vi "RWNoise-Init Stimulus.vi"(0 "RW Noise Params":T29, 7 "Expt State":T27, 11 "error in (no error)":errorcluster, 12 "RWN Stim":T28) -> (4 "Runtime":T1={"Stimulus"={"Waveform"={"Type"=enum."Tone", "Tone"={"Frequency (kHz)"=0.0, "Last Freq"=0.0, "Last Phase"=0.0}, "Pulse Train"={"Pulse width (us)"=0.0, "Pulse rate (Hz)"=0.0, "Gap (ms)"=0.0, "Polarity"=enum."POS", "PT State"={"Template"=[], "Nperiod"=0, "Index"=0, "Pulse Rate (Hz)"=0.0, "Phase (cycles)"=0.0, "Noff"=0}, "Asynch"=FALSE}, "Noise"={"InvFilt"=FALSE, "Noise"=[], "CurPt"=0, "Aweight"=FALSE, "Seed"=0, "afile"=path ""}, "File"={"Filename"=path "", "Signal"=[], "Channel"=0, "stream"=FALSE, "offset"=0, "nreps"=0, "loops"=0, "Randomize"=FALSE, "order"=[], "Seed"=0, "Tokens"=0}, "FMSweep"={"Rate (oct/s)"=0.0, "Fmin (Hz)"=0.0, "Fmax (Hz)"=0.0, "Ramp (ms)"=0.0, "Linear"=FALSE}, "Chirp Train"={"Params"={"Fmin (kHz)"=4.0, "Fmax (kHz)"=64.0, "Compensate"=FALSE, "Duration (ms)"=2.0}, "Data"={"WF"=[]}}, "Complex Tone"={"Params"={"F0 (Hz)"=0.0, "Band"={"Flow (Hz)"=0.0, "Fhigh (Hz)"=0.0}, "Phase"=enum."Cosine", "Min F0 (Hz)"=0.0, "Max F0 (Hz)"=0.0, "ContinRandPhase"=FALSE, "Max peak factor"=inf, "Max mod depth"=2.0, "MinHarmNum"=0, "MaxHarmNum"=0, "Level Mode"=enum."per component", "% jitter"=0.0}, "Data"={"Ncomp"=0, "MinHarm"=0, "Phase"=[], "Amplitude"=[], "Npts/frame"=0, "Last F0"=0.0, "Fmin"=0.0, "Fmax"=0.0, "Lslope"=0.0, "randphase"=FALSE, "overall rms"=FALSE, "fmult"=[], "jittered"=FALSE}}, "Moving Ripple"={"Params"={"Fmin"=0.0, "Fmax"=0.0, "Density"=0.0, "Velocity"=0.0, "Depth"=0.0, "Phase"=0.0, "Comp/oct"=0}, "Data"={"Freq"=[], "A"=[], "phase"=[], "Phase"=0.0}}}, "Filter"={"Type"=enum."Lowpass", "CF (kHz)"=0.0, "BW (kHz)"=0.0, "Cascade"=FALSE, "Quadrature"=FALSE, "Scale Factor"=0.0, "Stages"=[], "Class"=enum."Elliptic", "Order"=0, "BWUnits"=enum."Linear"}, "Burst"={"Active"=FALSE, "Delay (ms)"=0.0, "Duration (ms)"=0.0, "Ramp (ms)"=0.0, "Rate (Hz)"=0.0, "Trepeat (ms)"=0.0, "Repeat"=FALSE}, "Level"={"Level"=0.0, "Units"=enum."dB atten", "Max"=0.0, "Multiplier"=0.0, "Cal File"=path "", "Cal"={"Freq (Hz)"=[], "Mag (dB SPL)"=[], "Phase (deg)"=[]}}, "Name"="", "Advanced"={"Rep Mask"="", "AltPol"=FALSE, "Var"="", "Expr"="", "Persist"=FALSE}, "SAM"={"Active"=FALSE, "Frequency (Hz)"=0.0, "Depth"=0.0, "Init Phase (cycles)"=0.0, "phase (degrees)"=0.0, "Asynch"=FALSE}}, "Fs (Hz)"=0.0, "AO Npts"=0, "AO Channels"=[], "Active"=FALSE, "AINpts"=0, "WinPts"=0, "NUpdate"=0} {"Stimulus"."Filter"."Stages"."IIR Filter"."Forward Coefficients" format="%.4f"; "Stimulus"."Filter"."Stages"."IIR Filter"."Reverse Coefficients" format="%.4f"}, 8 "Coerced Freq (kHz)":dbl, 10 "Coerced pulse rate (Hz)":dbl, 15 "error out":errorcluster)   [LabVIEW 2020]
uses:
  RWNoise Params.ctl
  epl-vi-lib/Utility VIs/Type Defs/Left-Right ring.ctl
  RWNoise-Stim Params.ctl
  CFTS Main Panel SubVIs/CFTS-Experiment State.ctl
  epl-vi-lib/Signal Synthesis VIs/Controls/Stimulus Channel (Full)/Full Stimulus Channel Data.ctl
  epl-vi-lib/Signal Synthesis VIs/Controls/Waveform XCtl/Waveform Data.ctl
  epl-vi-lib/Signal Synthesis VIs/Controls/Waveform XCtl/Waveform Enum.ctl
  epl-vi-lib/Signal Synthesis VIs/Waveform VIs/Tone VIs/Tone Params.ctl
  epl-vi-lib/Signal Synthesis VIs/Waveform VIs/Pulse Train VIs/Pulse Train Params.ctl
  epl-vi-lib/Signal Synthesis VIs/Waveform VIs/Pulse Train VIs/Pulse Polarity.ctl
  epl-vi-lib/Signal Synthesis VIs/Waveform VIs/Pulse Train VIs/PT-Continuous State.ctl
  epl-vi-lib/Signal Synthesis VIs/Waveform VIs/Noise VIs/Noise Params.ctl
  epl-vi-lib/Signal Synthesis VIs/Waveform VIs/File VIs/StimFile-Params.ctl
  epl-vi-lib/Signal Synthesis VIs/Waveform VIs/FM Sweep VIs/FM Sweep Params.ctl
  epl-vi-lib/Signal Synthesis VIs/Waveform VIs/Chirp Train VIs/Chirp Train.ctl
  epl-vi-lib/Signal Synthesis VIs/Waveform VIs/Chirp Train VIs/Chirp Train Params.ctl
  epl-vi-lib/Signal Synthesis VIs/Waveform VIs/Complex Tone VIs/CT-Params.ctl
  epl-vi-lib/Signal Synthesis VIs/Waveform VIs/Complex Tone VIs/CT-Phase Enum.ctl
  epl-vi-lib/Signal Synthesis VIs/Waveform VIs/Complex Tone VIs/CT-Runtime Data.ctl
  epl-vi-lib/Signal Synthesis VIs/Waveform VIs/Moving Ripple VIs/Moving Ripple.ctl
  epl-vi-lib/Signal Synthesis VIs/Waveform VIs/Moving Ripple VIs/Moving Ripple.Params.ctl
  epl-vi-lib/Signal Synthesis VIs/Waveform VIs/Moving Ripple VIs/Moving Ripple.Data.ctl
  epl-vi-lib/Signal Synthesis VIs/Controls/Advanced Filter XCtl/Filter Data.ctl
  epl-vi-lib/Signal Synthesis VIs/Filter VIs/Filter-Bandwidth Units.ctl
  epl-vi-lib/Signal Synthesis VIs/Controls/Burst XCtl/Burst Data.ctl
  epl-vi-lib/Signal Synthesis VIs/Controls/Level XCtl/Level Data.ctl
  epl-vi-lib/Signal Synthesis VIs/Controls/Level XCtl/Level Units.ctl
  epl-vi-lib/Signal Synthesis VIs/Controls/Advanced Options XCtl/Advanced Stimulus Options.ctl
  epl-vi-lib/Signal Synthesis VIs/Modulation VIs/SAM VIs/SAM Params.ctl
  RWNoise-Runtime Data.ctl
  epl-vi-lib/Connection VIs/Type Defs/Output sources.ctl
  epl-vi-lib/Utility VIs/Type Defs/Speaker ring.ctl
  epl-vi-lib/Signal Synthesis VIs/Top Level VIs/Stimulus-Initialize (full).vi
  epl-vi-lib/Signal Synthesis VIs/Controls/Advanced Filter XCtl/Advanced Filter XCtl.xctl
  epl-vi-lib/Signal Synthesis VIs/Controls/Level XCtl/Level XCtl.xctl
  epl-vi-lib/Signal Synthesis VIs/Controls/Burst XCtl/Burst Control.xctl
  epl-vi-lib/Signal Synthesis VIs/Controls/Waveform XCtl/Waveform XCtl.xctl
  epl-vi-lib/Signal Synthesis VIs/Controls/Advanced Options XCtl/Advanced Stimulus Options.xctl
  epl-vi-lib/Signal Synthesis VIs/Controls/Stimulus Channel (Full)/Stimulus Channel (Full).xctl
panel:
  in  "Stimulus":T2={"Waveform"={"Type"=enum."Tone", "Tone"={"Frequency (kHz)"=0.0, "Last Freq"=0.0, "Last Phase"=0.0}, "Pulse Train"={"Pulse width (us)"=0.0, "Pulse rate (Hz)"=0.0, "Gap (ms)"=0.0, "Polarity"=enum."POS", "PT State"={"Template"=[], "Nperiod"=0, "Index"=0, "Pulse Rate (Hz)"=0.0, "Phase (cycles)"=0.0, "Noff"=0}, "Asynch"=FALSE}, "Noise"={"InvFilt"=FALSE, "Noise"=[], "CurPt"=0, "Aweight"=FALSE, "Seed"=0, "afile"=path ""}, "File"={"Filename"=path "", "Signal"=[], "Channel"=0, "stream"=FALSE, "offset"=0, "nreps"=0, "loops"=0, "Randomize"=FALSE, "order"=[], "Seed"=0, "Tokens"=0}, "FMSweep"={"Rate (oct/s)"=0.0, "Fmin (Hz)"=0.0, "Fmax (Hz)"=0.0, "Ramp (ms)"=0.0, "Linear"=FALSE}, "Chirp Train"={"Params"={"Fmin (kHz)"=4.0, "Fmax (kHz)"=64.0, "Compensate"=FALSE, "Duration (ms)"=2.0}, "Data"={"WF"=[]}}, "Complex Tone"={"Params"={"F0 (Hz)"=0.0, "Band"={"Flow (Hz)"=0.0, "Fhigh (Hz)"=0.0}, "Phase"=enum."Cosine", "Min F0 (Hz)"=0.0, "Max F0 (Hz)"=0.0, "ContinRandPhase"=FALSE, "Max peak factor"=inf, "Max mod depth"=2.0, "MinHarmNum"=0, "MaxHarmNum"=0, "Level Mode"=enum."per component", "% jitter"=0.0}, "Data"={"Ncomp"=0, "MinHarm"=0, "Phase"=[], "Amplitude"=[], "Npts/frame"=0, "Last F0"=0.0, "Fmin"=0.0, "Fmax"=0.0, "Lslope"=0.0, "randphase"=FALSE, "overall rms"=FALSE, "fmult"=[], "jittered"=FALSE}}, "Moving Ripple"={"Params"={"Fmin"=0.0, "Fmax"=0.0, "Density"=0.0, "Velocity"=0.0, "Depth"=0.0, "Phase"=0.0, "Comp/oct"=0}, "Data"={"Freq"=[], "A"=[], "phase"=[], "Phase"=0.0}}}, "Filter"={"Type"=enum."Lowpass", "CF (kHz)"=0.0, "BW (kHz)"=0.0, "Cascade"=FALSE, "Quadrature"=FALSE, "Scale Factor"=0.0, "Stages"=[], "Class"=enum."Elliptic", "Order"=0, "BWUnits"=enum."Linear"}, "Burst"={"Active"=FALSE, "Delay (ms)"=0.0, "Duration (ms)"=0.0, "Ramp (ms)"=0.0, "Rate (Hz)"=0.0, "Trepeat (ms)"=0.0, "Repeat"=FALSE}, "Level"={"Level"=0.0, "Units"=enum."dB atten", "Max"=0.0, "Multiplier"=0.0, "Cal File"=path "", "Cal"={"Freq (Hz)"=[], "Mag (dB SPL)"=[], "Phase (deg)"=[]}}, "Name"="", "Advanced"={"Rep Mask"="", "AltPol"=FALSE, "Var"="", "Expr"="", "Persist"=FALSE}, "SAM"={"Active"=FALSE, "Frequency (Hz)"=0.0, "Depth"=0.0, "Init Phase (cycles)"=0.0, "phase (degrees)"=0.0, "Asynch"=FALSE}} {"Filter"."Stages"."IIR Filter"."Forward Coefficients" format="%.4f"; "Filter"."Stages"."IIR Filter"."Reverse Coefficients" format="%.4f"}
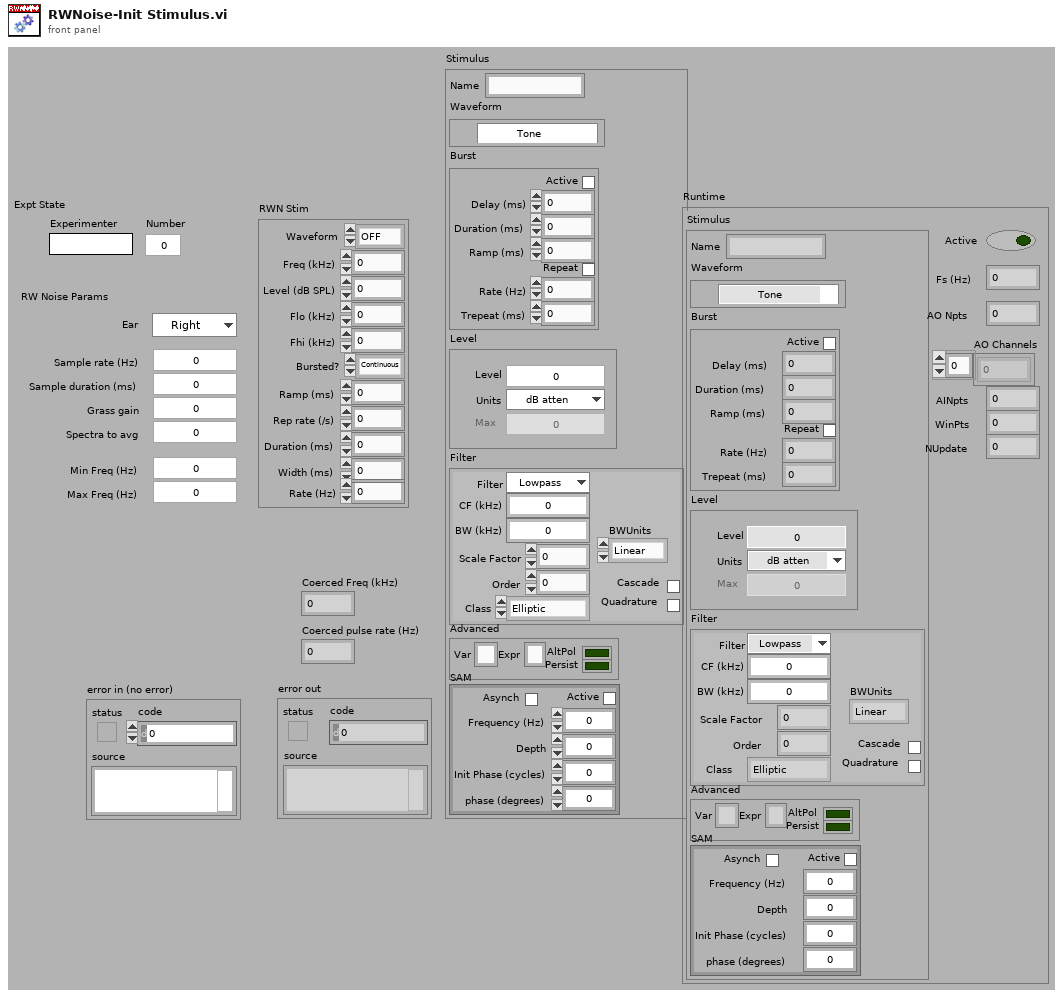
[diagram p1: front panel]
types:
  T1 = typedef "RWNoise-Runtime Data.ctl" = cluster{"Stimulus":T2, "Fs (Hz)":dbl, "AO Npts":i32, "AO Channels":i32[], "Active":bool, "AINpts":i32, "WinPts":i32, "NUpdate":i32}
  T2 = typedef "Stimulus Channel (Full).xctl/Full Stimulus Channel Data.ctl" = cluster{"Waveform":T3, "Filter":T20, "Burst":T22, "Level":T23, "Name":string, "Advanced":T25, "SAM":T26}
  T3 = typedef "Waveform XCtl.xctl/Waveform Data.ctl" = cluster{"Type":T4, "Tone":T5, "Pulse Train":T6, "Noise":T9, "File":T10, "FMSweep":T11, "Chirp Train":T12, "Complex Tone":cluster{"Params":T14, "Data":T16}, "Moving Ripple":T17}
  T4 = typedef "Waveform Enum.ctl" = enum16{"OFF", "Tone", "Noise", "Pulse Train", "File", "FM Sweep", "Chirp Train", "Complex Tone", "FM Tone", "Moving Ripple"}
  T5 = typedef "Tone Params.ctl" = cluster{"Frequency (kHz)":dbl, "Last Freq":dbl, "Last Phase":dbl}
  T6 = typedef "Pulse Train Params.ctl" = cluster{"Pulse width (us)":dbl, "Pulse rate (Hz)":dbl, "Gap (ms)":dbl, "Polarity":T7, "PT State":T8, "Asynch":bool}
  T7 = typedef "Pulse Polarity.ctl" = enum16{"POS", "NEG", "POS-NEG", "NEG-POS"}
  T8 = typedef "PT-Continuous State.ctl" = cluster{"Template":dbl[], "Nperiod":i32, "Index":i32, "Pulse Rate (Hz)":dbl, "Phase (cycles)":dbl, "Noff":i32}
  T9 = typedef "Noise Params.ctl" = cluster{"InvFilt":bool, "Noise":dbl[], "CurPt":i32, "Aweight":bool, "Seed":i32, "afile":path}
  T10 = typedef "StimFile-Params.ctl" = cluster{"Filename":path, "Signal":dbl[], "Channel":i32, "stream":bool, "offset":i32, "nreps":i32, "loops":i32, "Randomize":bool, "order":i32[], "Seed":i32, "Tokens":i32}
  T11 = typedef "FM Sweep Params.ctl" = cluster{"Rate (oct/s)":dbl, "Fmin (Hz)":dbl, "Fmax (Hz)":dbl, "Ramp (ms)":dbl, "Linear":bool}
  T12 = typedef "Chirp Train.ctl" = cluster{"Params":T13, "Data":cluster{"WF":dbl[]}}
  T13 = typedef "Chirp Train Params.ctl" = cluster{"Fmin (kHz)":dbl, "Fmax (kHz)":dbl, "Compensate":bool, "Duration (ms)":dbl}
  T14 = typedef "CT-Params.ctl" = cluster{"F0 (Hz)":dbl, "Band":cluster{"Flow (Hz)":dbl, "Fhigh (Hz)":dbl}, "Phase":T15, "Min F0 (Hz)":dbl, "Max F0 (Hz)":dbl, "ContinRandPhase":bool, "Max peak factor":dbl, "Max mod depth":dbl, "MinHarmNum":i32, "MaxHarmNum":i32, "Level Mode":enum16{"per component", "overall rms"}, "% jitter":dbl}
  T15 = typedef "CT-Phase Enum.ctl" = enum16{"Cosine", "Random", "Alternating"}
  T16 = typedef "CT-Runtime Data.ctl" = cluster{"Ncomp":i32, "MinHarm":i32, "Phase":dbl[], "Amplitude":dbl[], "Npts/frame":i32, "Last F0":dbl, "Fmin":dbl, "Fmax":dbl, "Lslope":dbl, "randphase":bool, "overall rms":bool, "fmult":dbl[], "jittered":bool}
  T17 = typedef "Moving Ripple.ctl" = cluster{"Params":T18, "Data":T19}
  T18 = typedef "Moving Ripple.Params.ctl" = cluster{"Fmin":dbl, "Fmax":dbl, "Density":dbl, "Velocity":dbl, "Depth":dbl, "Phase":dbl, "Comp/oct":i32}
  T19 = typedef "Moving Ripple.Data.ctl" = cluster{"Freq":dbl[], "A":dbl[], "phase":dbl[], "Phase":dbl}
  T20 = typedef "Advanced Filter XCtl.xctl/Filter Data.ctl" = cluster{"Type":enum16{"Lowpass", "Highpass", "Bandpass", "Bandstop", "OFF"}, "CF (kHz)":dbl, "BW (kHz)":dbl, "Cascade":bool, "Quadrature":bool, "Scale Factor":dbl, "Stages":cluster{"IIR Filter":cluster{"filter structure":enum32{"IIR 2nd Order", "IIR 4th Order"}, "Reverse Coefficients":dbl[], "Forward Coefficients":dbl[]}, "State":dbl[]}[], "Class":enum16{"Elliptic", "Butterworth"}, "Order":i32, "BWUnits":T21}
  T21 = typedef "Filter-Bandwidth Units.ctl" = enum16{"Linear", "Octaves", "Min-Max"}
  T22 = typedef "Burst Control.xctl/Burst Data.ctl" = cluster{"Active":bool, "Delay (ms)":dbl, "Duration (ms)":dbl, "Ramp (ms)":dbl, "Rate (Hz)":dbl, "Trepeat (ms)":dbl, "Repeat":bool}
  T23 = typedef "Level XCtl.xctl/Level Data.ctl" = cluster{"Level":dbl, "Units":T24, "Max":dbl, "Multiplier":dbl, "Cal File":path, "Cal":cluster{"Freq (Hz)":dbl[], "Mag (dB SPL)":dbl[], "Phase (deg)":dbl[]}}
  T24 = typedef "Level Units.ctl" = enum16{"dB atten", "dB SPL", "dB re 1 Vrms", "dB V/Hz½", "mW", "dB HL", "Volts", "dB mW"}
  T25 = typedef "Advanced Stimulus Options.xctl/Advanced Stimulus Options.ctl" = cluster{"Rep Mask":string, "AltPol":bool, "Var":string, "Expr":string, "Persist":bool}
  T26 = typedef "SAM Params.ctl" = cluster{"Active":bool, "Frequency (Hz)":dbl, "Depth":dbl, "Init Phase (cycles)":dbl, "phase (degrees)":dbl, "Asynch":bool}
  T27 = typedef "CFTS-Experiment State.ctl" = cluster{"Experimenter":string, "Number":u32, "Right":string, "Left":string, "Data Folder":path, "State File":path, "Version Info":string, "End Exposure Time":dbl, "Exposure Duration":string, "Run #":cluster{"CAP":i16, "ABR":i16, "DP":i16, "VsEP":i16, "MeasSeq":i16, "SubSeq":i16, "SFOAE":i16}}
  T28 = typedef "RWNoise-Stim Params.ctl" = cluster{"Waveform":enum16{"OFF", "Tone", "Noise", "Pulses"}, "Freq (kHz)":dbl, "Level (dB SPL)":dbl, "Flo (kHz)":dbl, "Fhi (kHz)":dbl, "Ramp (ms)":dbl, "Rep rate (/s)":dbl, "Bursted?":enum16{"Continuous", "Bursted"}, "Duration (ms)":dbl, "Width (ms)":dbl, "Rate (Hz)":dbl}
  T29 = typedef "RWNoise Params.ctl" = cluster{"Sample rate (Hz)":dbl, "Sample duration (ms)":dbl, "Grass gain":dbl, "Min Freq (Hz)":dbl, "Max Freq (Hz)":dbl, "Spectra to avg":i32, "Ear":T30}
  T30 = typedef "Left-Right ring.ctl" = enum16{"Right", "Left"}
  T31 = typedef "Speaker ring.ctl" = enum16{"Right primary", "Right secondary", "Left primary", "Left secondary"}
  T32 = typedef "Output sources.ctl" = u16
  T33 = enum16{"Lowpass", "Highpass", "Bandpass", "Bandstop", "OFF"}
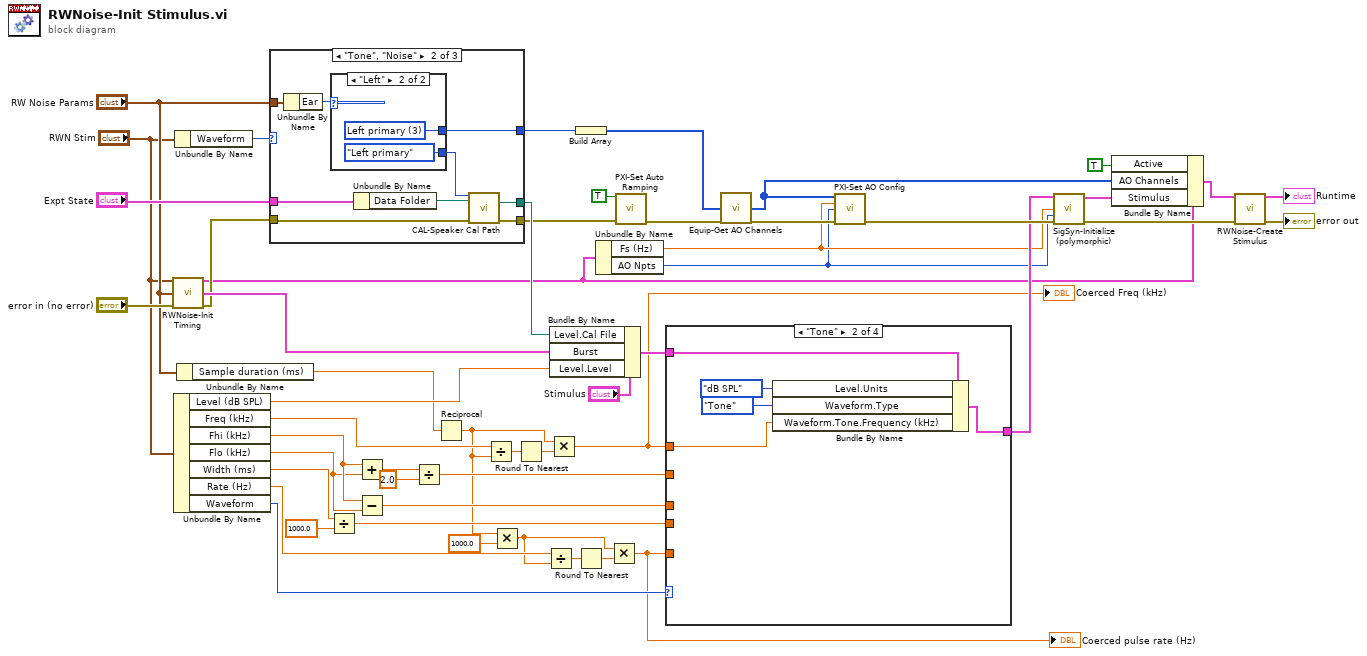
[diagram p0: block diagram]
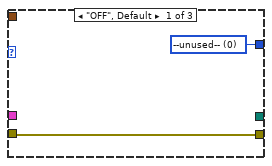
[diagram p2: hidden frame]
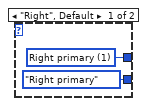
[diagram p3: hidden frame]
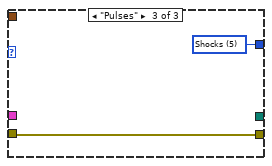
[diagram p4: hidden frame]
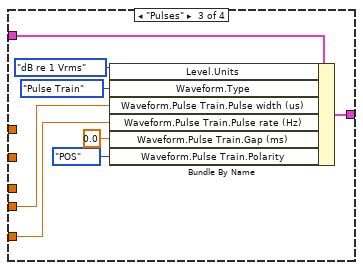
[diagram p6: hidden frame]
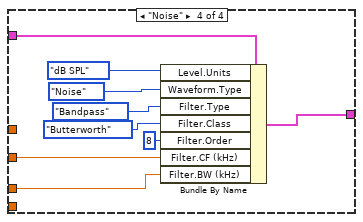
[diagram p7: hidden frame]
diagram:
  n1 = call "RWNoise-Init Timing.vi"("RWN Stim"="RWN Stim", "RW Noise Params"="RW Noise Params", "error in (no error)"="error in (no error)") -> ("Runtime"=w15:T1, "Burst Params"=w18:T22, "error out"=w17:errorcluster)  [unwired: 10 in]
  n2 = Unbundle By Name("RWN Stim") -> ("Level (dB SPL)"=w46:dbl, "Freq (kHz)"=w41:dbl, "Fhi (kHz)"=w36:dbl, "Flo (kHz)"=w35:dbl, "Width (ms)"=w10:dbl, "Rate (Hz)"=w5:dbl, "Waveform"=w21:enum16{"OFF", "Tone", "Noise", "Pulses"})
  n3 = Unbundle By Name("RWN Stim") -> ("Waveform"=w11:enum16{"OFF", "Tone", "Noise", "Pulses"})
  n4 = Unbundle By Name("RW Noise Params") -> ("Sample duration (ms)"=w20:dbl)
  n5 = case shown="\"Tone\", \"Noise\"" w11 {
    tunnel: [w53 w61 w68] -> w51
    tunnel: "Expt State" -> [_ w59 _]
    tunnel: [_ w57 _] -> w44
    tunnel: [w52 w56 w67] -> w31
    tunnel: w17 -> [w52 w55 w67]
    tunnel: "RW Noise Params" -> [_ w54 _]
    frame "OFF", Default {
      w53 = T32 0 items=["--unused--", "Right primary", "Right secondary", "Left primary", "Left secondary", "Shocks", "Startle", "Background", "Shaker"] ("Ring")
    }
    frame "Tone", "Noise" {
      n6 = Unbundle By Name(w54) -> ("Ear"=w62:T30)
      n7 = case shown="\"Left\"" w62 {
        tunnel: [w64 w66] -> w61
        tunnel: [Speaker_ring."Right primary" ("Speaker") Speaker_ring."Left primary" ("Speaker")] -> w60
        frame "Right", Default {
          w64 = T32 1 items=["--unused--", "Right primary", "Right secondary", "Left primary", "Left secondary", "Shocks", "Startle", "Background", "Shaker"] ("Ring")
        }
        frame "Left" {
          w66 = T32 3 items=["--unused--", "Right primary", "Right secondary", "Left primary", "Left secondary", "Shocks", "Startle", "Background", "Shaker"] ("Ring")
        }
      }
      n8 = Unbundle By Name(w59) -> ("Data Folder"=w58:path)
      n9 = call "CAL-Speaker Cal Path.vi"("Speaker"=w60, "Data Folder"=w58, "error in (no error)"=w55) -> ("Cal Path"=w57:path, "error out"=w56:errorcluster)  [unwired: 11 in]
    }
    frame "Pulses" {
      w68 = T32 5 items=["--unused--", "Right primary", "Right secondary", "Left primary", "Left secondary", "Shocks", "Startle", "Background", "Shaker"] ("Ring")
    }
  }
  n10 = Divide(x=w10, y=1000.0) -> (x/y=w8:dbl)
  n11 = Add(x=w36, y=w35) -> (x+y=w34:dbl)
  n12 = Subtract(x=w36, y=w35) -> (x-y=w37:dbl)
  n13 = Divide(x=w34, y=2.0) -> (x/y=w32:dbl)
  n14 = Reciprocal(x=w20) -> (1/x=w2:dbl)
  n15 = Divide(x=w41, y=w2) -> (x/y=w43:dbl)
  n16 = Multiply(x=w2, y=1000.0) -> (x*y=w3:dbl)
  n17 = Round To Nearest(number=w43) -> (nearest integer value=w42:dbl)
  n18 = Divide(x=w5, y=w3) -> (x/y=w7:dbl)
  n19 = Multiply(x=w2, y=w42) -> (x*y=w22:dbl)
  "Coerced Freq (kHz)" <- w22
  n20 = Bundle By Name(cluster="Stimulus", "Level.Cal File"=w44, "Burst"=w18, "Level.Level"=w46) -> (w40:T2)
  n21 = Build Array(w51) -> (w50:T32[])
  n22 = Round To Nearest(number=w7) -> (nearest integer value=w6:dbl)
  n23 = Unbundle By Name(w15) -> ("Fs (Hz)"=w14:dbl, "AO Npts"=w13:i32)
  n24 = Multiply(x=w3, y=w6) -> (x*y=w4:dbl)
  "Coerced pulse rate (Hz)" <- w4
  n25 = call "PXI-Set Auto Ramping.vi"("Auto ramp?"=TRUE, "error in (no error)"=w31) -> ("error out"=w30:errorcluster)  [unwired: 13 in]
  n26 = case shown="\"Tone\"" w21 {
    tunnel: w40 -> [w69 w74 w82 w91]
    tunnel: w22 -> [_ w71 _ _]
    tunnel: [w69 w72 w80 w89] -> w38
    tunnel: w37 -> [_ _ _ w87]
    tunnel: w32 -> [_ _ _ w86]
    tunnel: w4 -> [_ _ w76 _]
    tunnel: w8 -> [_ _ w75 _]
    frame "OFF", Default {
    }
    frame "Tone" {
      n27 = Bundle By Name(cluster=w74, "Level.Units"=Level_Units."dB SPL" ("Level.Mode"), "Waveform.Type"=Waveform_Enum."Tone", "Waveform.Tone.Frequency (kHz)"=w71) -> (w72:T2)
    }
    frame "Pulses" {
      n28 = Bundle By Name(cluster=w82, "Level.Units"=Level_Units."dB re 1 Vrms" ("Level.Mode"), "Waveform.Type"=Waveform_Enum."Pulse Train", "Waveform.Pulse Train.Pulse width (us)"=w75, "Waveform.Pulse Train.Pulse rate (Hz)"=w76, "Waveform.Pulse Train.Gap (ms)"=0.0, "Waveform.Pulse Train.Polarity"=Pulse_Polarity."POS") -> (w80:T2)
    }
    frame "Noise" {
      n29 = Bundle By Name(cluster=w91, "Level.Units"=Level_Units."dB SPL" ("Level.Mode"), "Waveform.Type"=Waveform_Enum."Noise", "Filter.Type"=T33."Bandpass", "Filter.Class"=enum16{"Elliptic", "Butterworth"}."Butterworth", "Filter.Order"=8, "Filter.CF (kHz)"=w86, "Filter.BW (kHz)"=w87) -> (w89:T2)
    }
  }
  n30 = call "Equip-Get AO Channels.vi"("Outputs"=w50, "error in (no error)"=w30) -> ("AO Channels"=w29:i32[], "error out"=w49:errorcluster)  [unwired: 12 in]
  n31 = call "PXI-Set AO Config.vi"("AO Channels"=w29, "Sampling Rate (Hz)"=w14, "Buffer Size"=w13, "error in (no error)"=w49) -> ("error out"=w39:errorcluster)  [unwired: 11 in]
  n32 = call-poly "SigSyn-Initialize (polymorphic).vi"("Stimulus Channel"=w38, "Sampling rate (Hz)"=w14, "Npts"=w13, "error in (no error)"=w39) -> ("Stimulus Channel out"=w28:T2, "error out"=w23:errorcluster)  [unwired: 9 in, 1 out]
  n33 = Bundle By Name(cluster=w15, "Active"=TRUE, "AO Channels"=w29, "Stimulus"=w28) -> (w26:T1)
  n34 = call "RWNoise-Create Stimulus.vi"("Runtime"=w26, "error in (no error)"=w23) -> ("Runtime Out"=→"Runtime":T1, "error out"=→"error out":errorcluster)  [unwired: 12 in]
